vi "CreateSTRING_FOR_LOGGING.vi"(11 "input DBL":dbl) -> (3 "String":string)   [LabVIEW 2016]
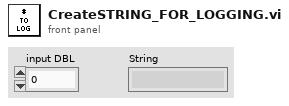
[diagram p1: front panel]
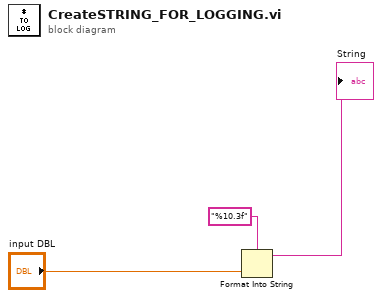
[diagram p0: block diagram]
diagram:
  n1 = Format Into String(format string="%10.3f", "input DBL") -> (resulting string=→"String":string)  [unwired: 2 in, 1 out]
